vi "Test Flatten SubClusters.vi"() -> ()   [LabVIEW 2017]
uses:
  06de8c1e-8f7f-4700-aedb-5029fcb6696e.vi
  7a335b94-5c49-4952-8c19-1b0d5863d5a5.vi
  Make JSON Object.vi
  JSON text to Variant (path).vi
  Find Item.vi
  String Subset.vi
  <vilib>/Utility/Data Type/Get Type Information.vi
  Variant to JSON Text.vi
  support/Format JSON Object.vi
  JSON text to Variant.vi
  Parsing/Parse Full Path or Item Name.vi
  Offset/Find Item Locations by Path.vi
  <vilib>/JDP Science/JDP Science Common Utilities/Array of Variants to Cluster.vi
  <vilib>/addons/_JKI Toolkits/Caraya/classes/Assert/Assert.lvclass
  <vilib>/addons/_JKI Toolkits/Caraya/classes/Test/Test.lvclass
panel:
  out "Cluster":T1
  out "<JSON>":string
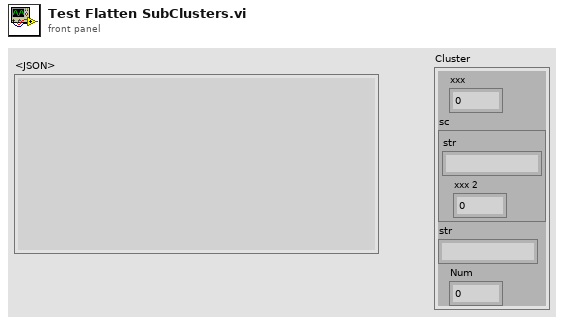
[diagram p1: front panel]
types:
  T1 = cluster{"xxx":i32, "sc":cluster{"str":string, "xxx 2":i32}, "str":string, "Num":i32}
  T2 = cluster{"xxx":i32, "sc":cluster{"Num":i32, "str":string}, "xxx 2":i32}
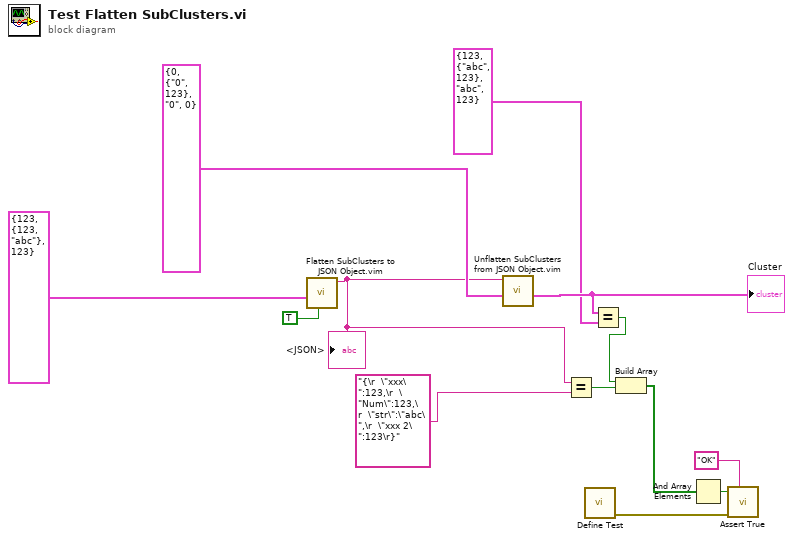
[diagram p0: block diagram]
diagram:
  n1 = call "Flatten SubClusters to JSON Object.vim"("Pretty Print?"=TRUE, "Any Cluster"=T2 {"xxx"=123, "sc"={"Num"=123, "str"="abc"}, "xxx 2"=123}) -> ("<JSON>"=w7:string)  [unwired: 8 in, 1 out]
  "<JSON>" <- w7
  n2 = call "Unflatten SubClusters from JSON Object.vim"("Any Cluster"=T1 {"xxx"=0, "sc"={"str"="0", "xxx 2"=123}, "str"="0", "Num"=0}, "JSON"=w7) -> ("Cluster"=w3:T1)  [unwired: 8 in, 1 out]
  "Cluster" <- w3
  n3 = Equal?(x=w7, y="{\r  \"xxx\":123,\r  \"Num\":123,\r  \"str\":\"abc\",\r  \"xxx 2\":123\r}" ("<JSON>")) -> (x = y?=w5:bool)
  n4 = call <vilib>:"Define Test.vi"() -> ("error out"=w9:errorcluster)  [unwired: 11 in]
  n5 = Equal?(x=w3, y=T1 {"xxx"=123, "sc"={"str"="abc", "xxx 2"=123}, "str"="abc", "Num"=123} ("Cluster")) -> (x = y?=w1:bool)
  n6 = Build Array(w1, w5) -> (w4:bool[])
  n7 = And Array Elements(Boolean array=w4) -> (logical AND=w11:bool)
  n8 = call <vilib>:"Assert True.vi"("Label"="OK", "error in (no error)"=w9, "True?"=w11) -> ()  [unwired: 8 in, 1 out]
